vi "fw103_with_subvi_setandmove_errorhandle_noinit.vi"(0 "Device reference input":refnum<k24>, 5 "Method reference input":refnum<k24>, 7 "Set position\n(deg) (float)":dbl, 9 "Move (bool)":bool, 11 "Set/Move":dbl, 13 "Stop all (bool)":bool) -> (4 "Device reference out":refnum<k24>, 6 "Method reference out":refnum<k24>, 15 "Current position (deg) (float)":i32 format="%.3f")   [LabVIEW 2020]
uses:
  C:/Users/OPMuser/Documents/labview/fw103/Thorlabs.MotionControl.Benchtop.StepperMotorCLI.dll
  Thorlabs.MotionControl.Benchtop.StepperMotorCLI.dll
  C:/Users/OPMuser/Documents/labview/fw103/Thorlabs.MotionControl.Controls.dll
  Thorlabs.MotionControl.Controls.dll
  <extravilib>/ChannelInstances/Stream-bool/Read With Abort.vi
  <extravilib>/ChannelInstances/Tag-bool/Write With Abort.vi
  <extravilib>/ChannelInstances/Tag-bool/Read With Abort.vi
  <extravilib>/ChannelInstances/Stream-bool/Write With Abort.vi
  <extravilib>/ChannelInstances/Stream-bool/EndpointRead.vi
  <extravilib>/ChannelInstances/Stream-bool/Endpoint.vi
  <extravilib>/ChannelInstances/Stream-bool/Instantiate.vi
  <extravilib>/ChannelInstances/Tag-bool/Instantiate.vi
  <extravilib>/ChannelInstances/Stream-bool/)Channel.vi
  <resource>/ChannelSupport/_ChannelSupport/WaitIfNeeded.vi
  <vilib>/Utility/error.llb/Error Cluster From Error Code.vi
  <extravilib>/ChannelInstances/Tag-bool/Endpoint.vi
  <extravilib>/ChannelInstances/Tag-bool/EndpointRead.vi
  <vilib>/ErrorRing/Error Ring.xnode
  <extravilib>/ChannelInstances/Tag-bool.lvlib
  <extravilib>/ChannelInstances/Stream-bool.lvlib
panel:
  # "Filter wheel control"
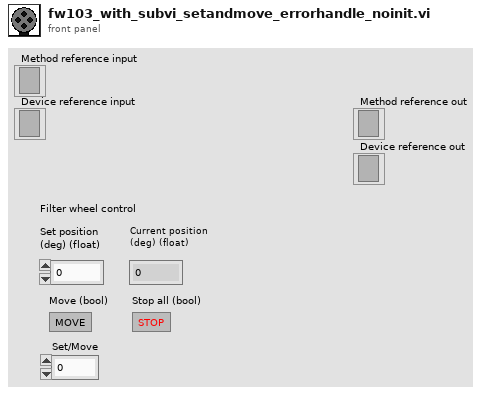
[diagram p1: front panel]
types:
  T1 = typedef "Tag-bool.lvlib/))Channel.ctl" = refnum<queue>
  T2 = typedef "Stream-bool.lvlib/)Channel.ctl" = refnum<queue>
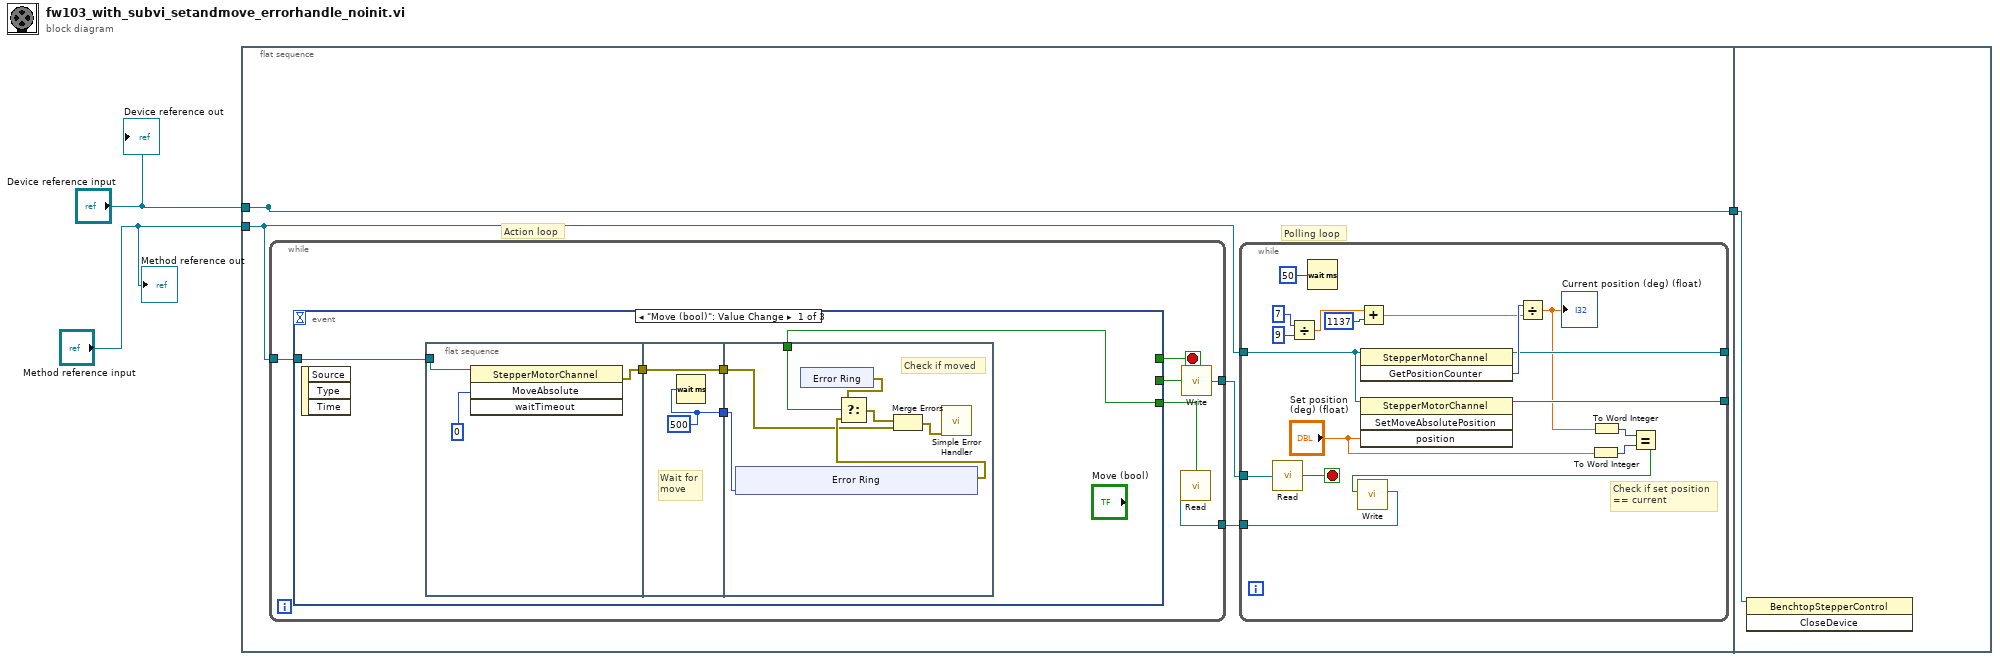
[diagram p0: block diagram]
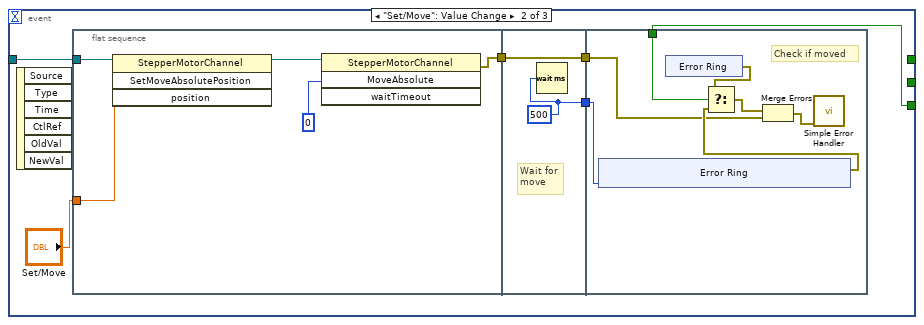
[diagram p2: hidden frame]
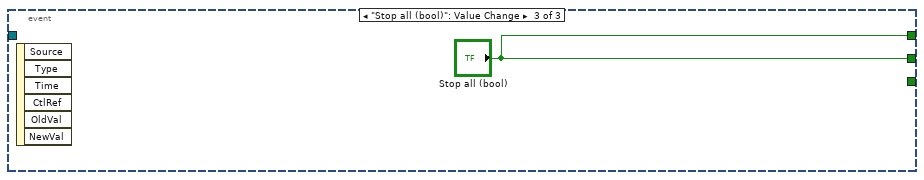
[diagram p3: hidden frame]
diagram:
  n1 = flat-sequence {
    tunnel: [w4] -> _
    tunnel: [w4] -> w3
    tunnel: "Method reference input" -> [w5]
    tunnel: "Device reference input" -> [w4]
    tunnel: w3 -> [w86]
    frame #0 {
      # "Action loop"
      # "Polling loop"
      n2 = while {
        tunnel: [w11] -> w7
        tunnel: w5 -> [w10]
        tunnel: w6 -> [w8]
        stop <- w13 stop-if-true
        n3 = call <extravilib>:"Read.vi"("channel"=w8) -> ("element"=w9:bool)  [unwired: 6 in, 4 out]
        n4 = event shown="[0] \"Move (bool)\": Value Change" {
          selector: _ -> [_ _ _]
          dyn-events: _ -> [_ _ _]
          timeout: _ -> [_ _ _]
          tunnel: [_ _ "Stop all (bool)"] -> w13
          tunnel: [_ _ "Stop all (bool)"] -> w12
          tunnel: w10 -> [w14 w41 _]
          tunnel: w9 -> [w17 w40 _]
          event "Move (bool)": Value Change {
            n5 = event-data() -> ()  [unwired: 1 in, 3 out]
            n6 = flat-sequence {
              tunnel: w14 -> [w20]
              tunnel: [w19] -> w15
              tunnel: [w23] -> w18
              tunnel: [w22] -> w16
              tunnel: w15 -> [w22]
              tunnel: w18 -> [w30]
              tunnel: w17 -> [w29]
              tunnel: w16 -> [w25]
              frame #0 {
                n7 = invoke class="StepperMotorChannel" method="MoveAbsolute"(reference=w20, "waitTimeout"=0) -> (error out=w19:errorcluster)  [unwired: 2 in, 3 out]
              }
              frame #1 {
                w23 = 500 ("waitTimeout")
                # "Wait for\nmove"
                n8 = Wait (ms)(milliseconds to wait=w23) -> ()  [unwired: 1 out]
              }
              frame #2 {
                # "Check if moved"
                n9 = xnode "Error Ring"("parameter 0"=w30) -> ("error out"=w27:errorcluster)
                n10 = xnode "Error Ring"() -> ("error out"=w28:errorcluster)
                n11 = Select(t=w28, s=w29, f=w27) -> (s? t:f=w26:errorcluster)
                n12 = Merge Errors(w26, w25) -> (w24:errorcluster)
                n13 = call <vilib>:"Simple Error Handler.vi"("error in (no error)"=w24) -> ()  [unwired: 4 in, 5 out]
              }
            }
          }
          event "Set/Move": Value Change {
            n14 = event-data() -> ()  [unwired: 1 in, 6 out]
            n15 = flat-sequence {
              tunnel: [w48] -> w44
              tunnel: "Set/Move" -> [w47]
              tunnel: w41 -> [w46]
              tunnel: [w51] -> w43
              tunnel: [w50] -> w42
              tunnel: w44 -> [w50]
              tunnel: w43 -> [w58]
              tunnel: w40 -> [w57]
              tunnel: w42 -> [w53]
              frame #0 {
                n16 = invoke class="StepperMotorChannel" method="SetMoveAbsolutePosition"(reference=w46, "position"=w47) -> (reference out=w45:refnum<k24>)  [unwired: 2 in, 3 out]
                n17 = invoke class="StepperMotorChannel" method="MoveAbsolute"(reference=w45, "waitTimeout"=0) -> (error out=w48:errorcluster)  [unwired: 2 in, 3 out]
              }
              frame #1 {
                w51 = 500 ("waitTimeout")
                # "Wait for\nmove"
                n18 = Wait (ms)(milliseconds to wait=w51) -> ()  [unwired: 1 out]
              }
              frame #2 {
                # "Check if moved"
                n19 = xnode "Error Ring"("parameter 0"=w58) -> ("error out"=w55:errorcluster)
                n20 = xnode "Error Ring"() -> ("error out"=w56:errorcluster)
                n21 = Select(t=w56, s=w57, f=w55) -> (s? t:f=w54:errorcluster)
                n22 = Merge Errors(w54, w53) -> (w52:errorcluster)
                n23 = call <vilib>:"Simple Error Handler.vi"("error in (no error)"=w52) -> ()  [unwired: 4 in, 5 out]
              }
            }
          }
          event "Stop all (bool)": Value Change {
            n24 = event-data() -> ()  [unwired: 1 in, 6 out]
          }
        }
        n25 = call <extravilib>:"Write.vi"("element"=w12) -> ("channel"=w11:T1)  [unwired: 1 out]
      }
      n26 = while {
        tunnel: w5 -> [w77]
        tunnel: [w78] -> _
        tunnel: [w74] -> _
        tunnel: w7 -> [w76]
        tunnel: [w68] -> w6
        stop <- w75 stop-if-true
        # "Check if set position\n== current"
        n27 = call <extravilib>:"Read.vi"("channel"=w76) -> ("element"=w75:bool)  [unwired: 1 in, 1 out]
        n28 = Divide(x=7, y=9) -> (x/y=w81:dbl)
        n29 = Wait (ms)(milliseconds to wait=u32 50) -> ()  [unwired: 1 out]
        n30 = Add(x=w81, y=1137) -> (x+y=w79:dbl)
        n31 = invoke class="StepperMotorChannel" method="GetPositionCounter"(reference=w77) -> (reference out=w78:refnum<k24>, "GetPositionCounter"=w82:i32)  [unwired: 2 in, 1 out]
        n32 = invoke class="StepperMotorChannel" method="SetMoveAbsolutePosition"(reference=w77, "position"="Set position\n(deg) (float)") -> (reference out=w74:refnum<k24>)  [unwired: 2 in, 3 out]
        n33 = Divide(x=w82, y=w79) -> (x/y=w73:dbl)
        "Current position (deg) (float)" <- w73
        n34 = To Word Integer(number="Set position\n(deg) (float)") -> (16bit integer=w70:i16)
        n35 = To Word Integer(number=w73) -> (16bit integer=w71:i16)
        n36 = Equal?(x=w71, y=w70) -> (x = y?=w69:bool)
        n37 = call <extravilib>:"Write.vi"("element"=w69) -> ("channel"=w68:T2)  [unwired: 8 in, 2 out]
      }
    }
    frame #1 {
      n38 = invoke class="BenchtopStepperControl" method="CloseDevice"(reference=w86) -> ()  [unwired: 2 in, 3 out]
    }
  }
  "Method reference out" <- "Method reference input"
  "Device reference out" <- "Device reference input"
